vi "TargetHold.vi"(0 "DO Task":refnum<k21>="BlueSimple_DO_All", 1 "Touch lines":T1={"Home touch"=0, "Touch 1"=1, "Touch 2"=2, "Touch 3"=3, "Touch 4"=4}, 2 "DI Task":refnum<k21>, 5 "target hold":cluster{"Fix":dbl, "Rnd":dbl}={"Fix"=0.5, "Rnd"=0.5} {"Rnd" format="%.4f"; "Fix" format="%.4f"}, 7 "Home+target OK?":bool, 9 "target\nbounce-off":cluster{"Fix":dbl, "Rnd":dbl}={"Fix"=0.3, "Rnd"=0.0} caption="Allowed\nbounce-off" {"Rnd" format="%.4f"; "Fix" format="%_4g"}, 11 "Target":i16, 12 "Post-capture brightness":i16 caption="Brightness", 14 "Initialize?":bool) -> (4 "Go to stage":T2(ring), 15 "Last trial successful?":bool)   [LabVIEW 2010]
panel:
  # "+"
  # "+"
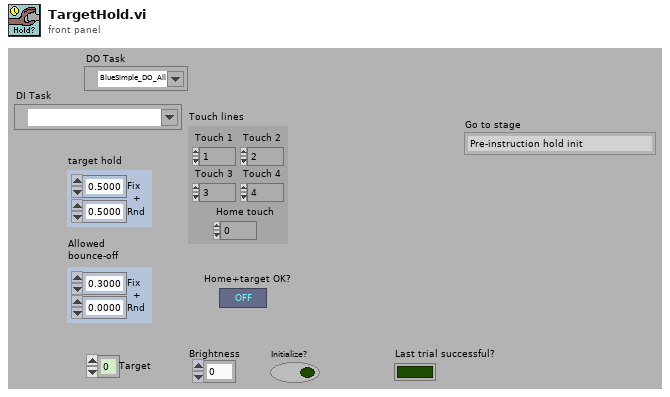
[diagram p1: front panel]
types:
  T1 = cluster{"Home touch":i16, "Touch 1":i16, "Touch 2":i16, "Touch 3":i16, "Touch 4":i16}
  T2 = enum16{"Pre-instruction hold init", "Pre-instruction hold", "Instruction init", "Instruction", "Post-instruction hold init", "Post-instruction hold", "Target capture init", "Target capture", "Target hold init", "Target hold", "Reward stage", "Intertrial"}
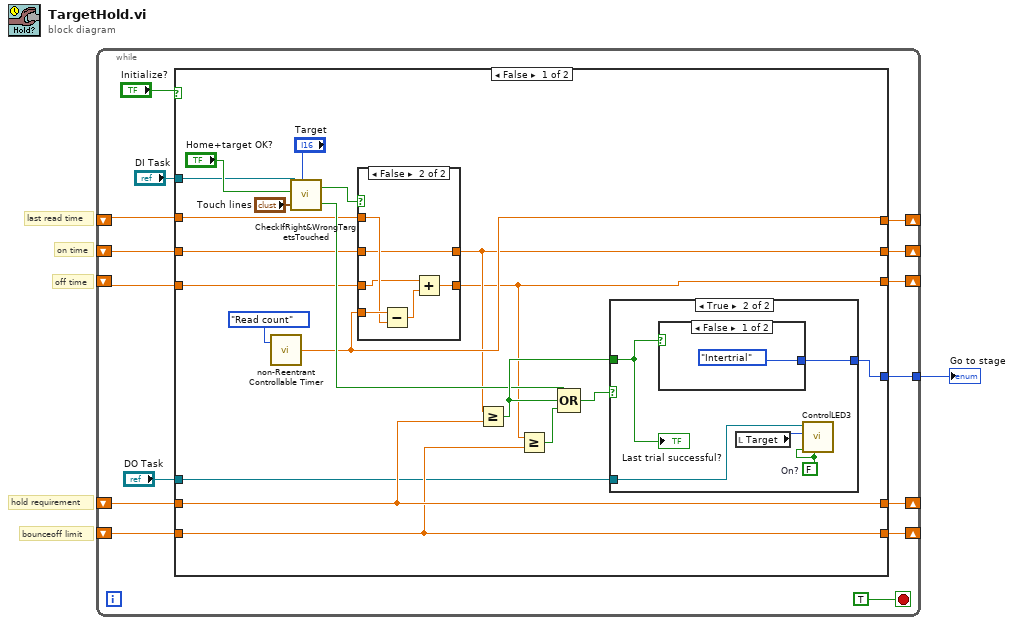
[diagram p0: block diagram]
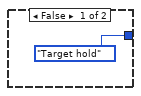
[diagram p2: hidden frame]
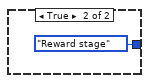
[diagram p3: hidden frame]
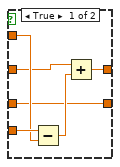
[diagram p4: hidden frame]
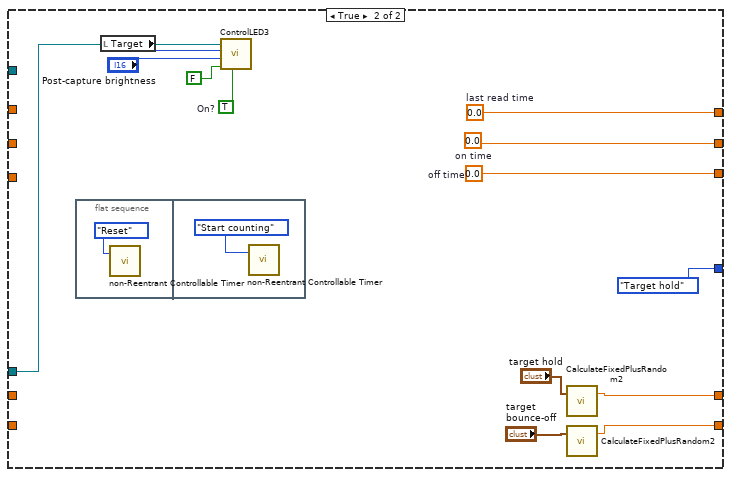
[diagram p5: hidden frame]
diagram:
  # "bounceoff limit"
  # "hold requirement"
  # "off time"
  # "on time"
  # "last read time"
  n1 = while {
    tunnel: [w15] -> w1
    shift-right: [w13] -> _
    shift-left: _ -> [w10]
    shift-right: [w12] -> _
    shift-left: _ -> [w9]
    shift-right: [w11] -> _
    shift-left: _ -> [w8]
    shift-right: [w7] -> _
    shift-left: _ -> [w5]
    shift-right: [w6] -> _
    shift-left: _ -> [w4]
    stop <- TRUE stop-if-true
    n2 = case shown="False" "Initialize?" {
      tunnel: [w36 T2."Target hold" ("Current stage")] -> w15
      tunnel: [w26 w69] -> w13
      tunnel: [w25 w68] -> w12
      tunnel: [w24 w67] -> w11
      tunnel: w10 -> [w29 _]
      tunnel: w9 -> [w28 _]
      tunnel: w8 -> [w27 _]
      tunnel: [w22 w63] -> w7
      tunnel: [w21 w62] -> w6
      tunnel: w5 -> [w22 _]
      tunnel: w4 -> [w21 _]
      tunnel: "DO Task" -> [w18 w57]
      tunnel: "DI Task" -> [w17 _]
      frame False {
        n3 = call "non-Reentrant Controllable Timer.vi"("Enum"=enum16{"Start counting", "Read count", "Reset"}."Read count") -> ("Time out"=w26:dbl)  [unwired: 1 in]
        n4 = call "CheckIfRight&WrongTargetsTouched.vi"("Target"="Target", "Touch sensor lines"="Touch lines", "Home+target OK?"="Home+target OK?", "DI Task"=w17) -> ("Wrong target touched?"=w31:bool, "Target touched?"=w33:bool)  [unwired: 2 in]
        n5 = case shown="False" w33 {
          tunnel: w28 -> [w45 w54]
          tunnel: w27 -> [w47 w51]
          tunnel: w26 -> [w49 w56]
          tunnel: w29 -> [w48 w55]
          tunnel: [w47 w53] -> w24
          tunnel: [w46 w54] -> w25
          frame True {
            n6 = Subtract(x=w49, y=w48) -> (x-y=w50:dbl)
            n7 = Add(x=w45, y=w50) -> (x+y=w46:dbl)
          }
          frame False {
            n8 = Subtract(x=w56, y=w55) -> (x-y=w52:dbl)
            n9 = Add(x=w51, y=w52) -> (x+y=w53:dbl)
          }
        }
        n10 = Greater Or Equal?(x=w25, y=w22) -> (x >= y?=w35:bool)
        n11 = Greater Or Equal?(x=w24, y=w21) -> (x >= y?=w32:bool)
        n12 = Compound Arithmetic op=OR(w31, w35, w32) -> (w23:bool)
        n13 = case shown="True" w23 {
          tunnel: [T2."Target hold" ("Current stage") w42] -> w36
          tunnel: w35 -> [_ w41]
          tunnel: w18 -> [_ w38]
          frame False {
          }
          frame True {
            w39 = FALSE  # On?
            n14 = case shown="False" w41 {
              tunnel: [T2."Intertrial" ("Current stage") T2."Reward stage" ("Current stage")] -> w42
              frame False {
              }
              frame True {
              }
            }
            n15 = local read "Target"() -> (w40:i16)
            n16 = call "ControlLED3.vi"("On?"=w39, "All flash?"=w39, "Target"=w40, "DO Task"=w38) -> ()  [unwired: 7 in]
            "Last trial successful?" <- w41
          }
        }
      }
      frame True {
        w61 = TRUE  # On?
        w69 = 0.0  # last read time
        w67 = 0.0  # off time
        w68 = 0.0  # on time
        n17 = flat-sequence {
          frame #0 {
            n18 = call "non-Reentrant Controllable Timer.vi"("Enum"=enum16{"Start counting", "Read count", "Reset"}."Reset") -> ()  [unwired: 1 in, 1 out]
          }
          frame #1 {
            n19 = call "non-Reentrant Controllable Timer.vi"("Enum"=enum16{"Start counting", "Read count", "Reset"}."Start counting") -> ()  [unwired: 1 in, 1 out]
          }
        }
        n20 = local read "Target"() -> (w59:i16)
        n21 = call "ControlLED3.vi"("On?"=w61, "All flash?"=FALSE, "Brightness"="Post-capture brightness", "Target"=w59, "DO Task"=w57) -> ()  [unwired: 6 in]
        n22 = call "CalculateFixedPlusRandom2.vi"("Component times"="target hold") -> ("Composite time"=w63:dbl)  [unwired: 1 in, 1 out]
        n23 = call "CalculateFixedPlusRandom2.vi"("Component times"="target\nbounce-off") -> ("Composite time"=w62:dbl)  [unwired: 1 in, 1 out]
      }
    }
  }
  "Go to stage" <- w1
